vi "1-search array.vi"() -> ()   [LabVIEW 2018]
panel:
  in  "element":i32
  out "index of element":i32
  in  "Array":i32[](array[numeric])
  # "This program uses function SEARCH 1D ARRAY"
  # "gives out -1 for the elements\nthat are not present in the array"
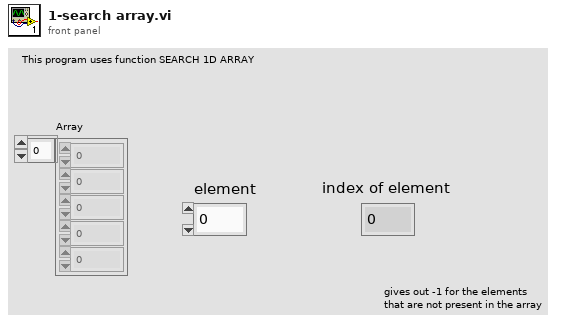
[diagram p1: front panel]
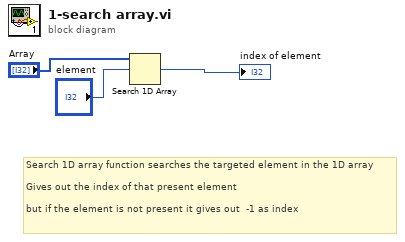
[diagram p0: block diagram]
diagram:
  # "Search 1D array function searches the targeted element in the 1D array\n \nGives out the index of that present element \n\nbut if the element is not present it gives out  -1 as index"
  n1 = Search 1D Array(1D array="Array", element="element") -> (index of element=→"index of element":i32)  [unwired: 1 in]
